vi "BB Vref Test.vi"(11 "Board Selector":T1) -> (0 "Error Out":errorcluster[](array[cluster]), 3 "Voltage Readings":dbl[](array[numeric]))   [LabVIEW 2022 SP3]
uses:
  Serial Board Com/Board Select.ctl
  Serial Board Com/ADCSelector BB.ctl
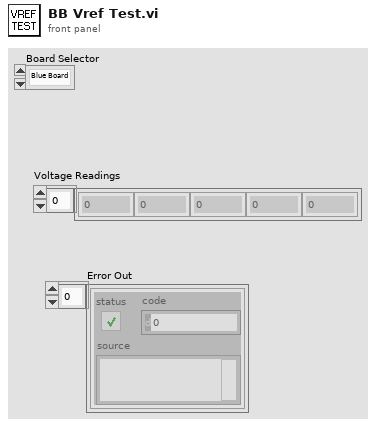
[diagram p1: front panel]
types:
  T1 = typedef "Board Select.ctl" = enum16{"Blue Board", "Green Board"}
  T2 = typedef "ADCSelector BB.ctl" = enum16{"INVA_ISENSE_U", "INVA_ISENSE_V", "INVA_ISENSE_W", "INVA_UDC", "INVA_TEMP", "HB_TEMP", "AUXB_TEMP", "VLINE_AB", "VLINE_BC", "VLINE_CA", "VSENSE_POS_24V", "VSENSE_POS_5V", "VSENSE_NEG_15V", "INVB_ISENSE_U", "INV_B_ISENSEV", "INVB_ISENSE_W", "INVB_UDC", "INVB_TEMP", "AUXA_TEMP", "AUXC_TEMP", "VOUT_AB", "VOUT_BC", "VOUT_CA", "VSENSE_POS_15V", "VSENSE_POS_3P3V", "TEST_POINT"}
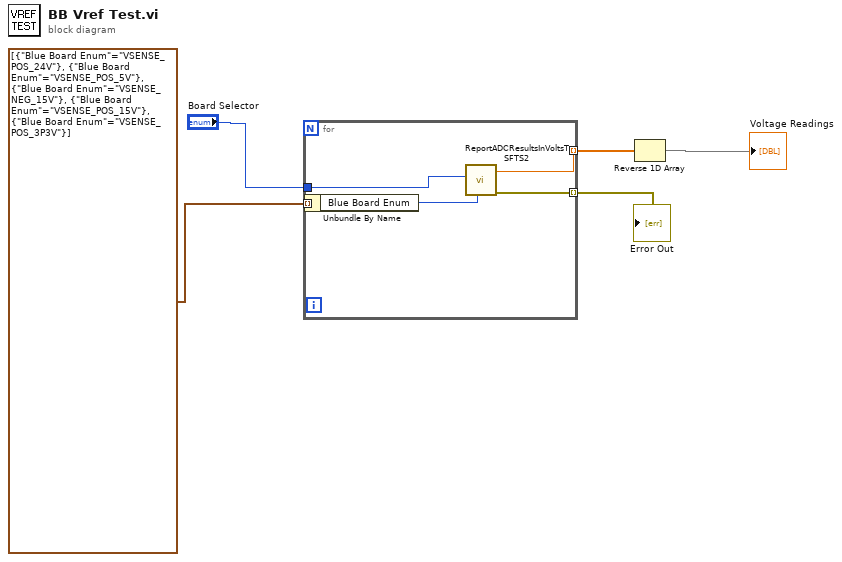
[diagram p0: block diagram]
diagram:
  n1 = for {
    tunnel: [w10] -> w5 mode=indexing
    tunnel: [w9] -> w3 mode=indexing
    tunnel: cluster{"Blue Board Enum":T2}[] [{"Blue Board Enum"=enum."VSENSE_POS_24V"}, {"Blue Board Enum"=enum."VSENSE_POS_5V"}, {"Blue Board Enum"=enum."VSENSE_NEG_15V"}, {"Blue Board Enum"=enum."VSENSE_POS_15V"}, {"Blue Board Enum"=enum."VSENSE_POS_3P3V"}] -> [w8] mode=indexing
    tunnel: "Board Selector" -> [w7]
    n2 = Unbundle By Name(w8) -> ("Blue Board Enum"=w6:T2)
    n3 = call "ReportADCResultsInVoltsTSFTS2.vi"("Blue Board Enum"=w6, "Board Selector"=w7) -> ("error out"=w9:errorcluster, "Result"=w10:dbl)  [unwired: 6 in, 2 out]
  }
  "Error Out" <- w3
  n4 = Reverse 1D Array(array=w5) -> (reversed array=→"Voltage Readings":dbl[])
